vi "RGB LED - Rainbow Pin 8 70 LEDs.vi"   [LabVIEW 2015]
doc: "This example demonstrates a rainbow effect on a 1-wire RGB LED strip using a WS2811 or WS2812 controller. Each LED in the strip is gradually changed from red to green, then to blue with a blend of colors in between. The LED color changing effect is staggered down the strip so not all LEDs are changed at the same time. The time delay can also be adjusted to change how fast the color is changed."
uses:
  <vilib>/Aledyne-TSXperts/Arduino Compatible Compiler for LabVIEW/Code Generator/Arduino APIs/RGB LED Strip/RGB Strip Mode.ctl
  <vilib>/Aledyne-TSXperts/Arduino Compatible Compiler for LabVIEW/Arduino Compatible Compiler for LabVIEW.lvlib
panel:
  # "Overview: Demonstrates a rainbow effect on a 1-wire RGB LED strip using a WS2811 or WS2812 controller.  Each LED in the strip is gradually changed from red to green, then to blue with a blend of colors in between.  The LED color changing effect is staggered down the strip so not all LEDs are changed at the same time.  The time delay can also be adjusted to change how fast the color is changed.\n\nInstructions:\n1. Wire a 1-wire LED strip to a digital pin on the Arduino board.  Follow wiring instructions from the manufacturer.  A 100-500 ohm resistor is usually recommended between the Arduino digital output and the LED strip's data in pin.  Also, a 100 uF capacitor between the ground and power input may reduce noise on from the power supply.  It is also recommended to power the LED strip from a separate power input if available on the strip.  When daisy chaining LED strips, it is recommended to only daisy chain the Data line and to power each strip from a separate power input.\n2. Set the Digital Pin wired below.\n3. Set the Mode to the correct setting for your LED strip (the WS2812 uses 800kHz GRB).\n4. Set the Number of LEDs on your strip.  This can be set to any number equal to or smaller than the number of physical LEDs on the strip of you do not wish to power up all of them.\n5. Set the delay (ms) between changes to the LED color.\n6.  If this example has been loaded from the Arduino Compatible Compiler for LabVIEW, simply select Compile and Download.  Otherwise, open Tools>Arduino Compatible Compiler for LabVIEW in LabVIEW, then select File>Load VI, and select this VI and then Compile and Download.\n7. Observe the LEDs on the strip changing color with a seamless rainbow transition."
types:
  T1 = typedef "Arduino Compatible Compiler for LabVIEW.lvlib/RGB Strip Mode.ctl" = u16
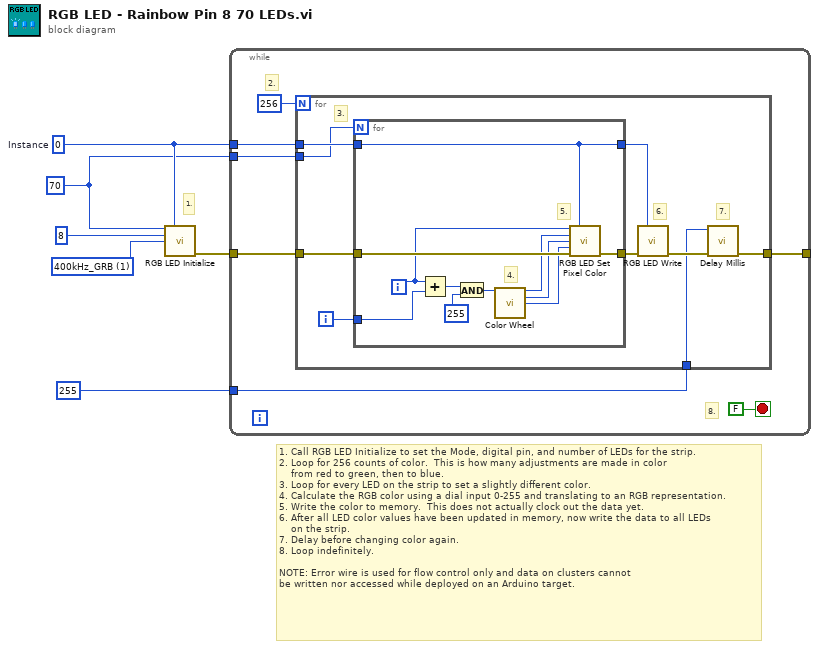
[diagram p0: block diagram]
diagram:
  w2 = u16 70 ("Number of LEDs")
  w6 = T1 1 items=["400kHz_RGB"=0, "400kHz_GRB"=1, "400kHz_BRG"=4, "800kHz_RGB"=2, "800kHz_GRB"=3, "400kHz_BRG"=6] ("Mode")
  w3 = u8 0  # Instance
  # "1."
  # "1. Call RGB LED Initialize to set the Mode, digital pin, and number of LEDs for the strip.\n2. Loop for 256 counts of color.  This is how many adjustments are made in color\n    from red to green, then to blue.\n3. Loop for every LED on the strip to set a slightly different color.\n4. Calculate the RGB color using a dial input 0-255 and translating to an RGB representation.\n5. Write the color to memory.  This does not actually clock out the data yet.\n6. After all LED color values have been updated in memory, now write the data to all LEDs\n    on the strip.\n7. Delay before changing color again.\n8. Loop indefinitely.\n\nNOTE: Error wire is used for flow control only and data on clusters cannot\nbe written nor accessed while deployed on an Arduino target."
  n1 = call <vilib>:"RGB LED Initialize.vi"("Number of Pixels"=w2, "Instance"=w3, "Pin"=u8 8 ("Digital Pin"), "Mode"=w6) -> ("error out"=w4:errorcluster)  [unwired: 11 in]
  n2 = while {
    tunnel: w4 -> [w11]
    tunnel: w3 -> [w9]
    tunnel: w2 -> [w10]
    tunnel: u8 255 ("delay (ms)") -> [w7]
    tunnel: [w8] -> _
    stop <- FALSE stop-if-true
    # "2."
    # "8."
    n3 = for {
      N: u16 256 ("Number of Pixels") -> [_]
      tunnel: w9 -> [w22]
      tunnel: w10 -> [w17]
      tunnel: w11 -> [w16]
      tunnel: [w15] -> w8
      tunnel: w7 -> [w14]
      i -> [w21]
      # "7."
      # "6."
      # "3."
      n4 = for {
        N: w17 -> [_]
        tunnel: w22 -> [w23]
        tunnel: w16 -> [w29]
        tunnel: w21 -> [w33]
        tunnel: [w24] -> w19
        tunnel: [w23] -> w18
        i -> [w25]
        # "5."
        # "4."
        n5 = Add(x=w25, y=w33) -> (x+y=w32:i32)
        n6 = And(x=w32, y=u8 255) -> (x .and. y?=w30:i32)
        n7 = call "Color Wheel.vi"("Dial Position"=w30) -> ("Red"=w28:u8, "Green"=w27:u8, "Blue"=w26:u8)  [unwired: 12 in]
        n8 = call <vilib>:"RGB LED Set Pixel Color.vi"("Pixel"=w25, "Instance"=w23, "Red"=w28, "Green"=w27, "Blue"=w26, "error in (no error)"=w29) -> ("error out"=w24:errorcluster)  [unwired: 9 in]
      }
      n9 = call <vilib>:"RGB LED Write.vi"("Instance"=w18, "error in (no error)"=w19) -> ("error out"=w20:errorcluster)  [unwired: 13 in]
      n10 = call <vilib>:"Delay Millis.vi"("error in (no error)"=w20, "delay"=w14) -> ("error out"=w15:errorcluster)  [unwired: 9 in]
    }
  }
